vi "DAC Run.vi"(8 "error in":errorcluster, 11 "DAC HeatFlow Temp in":refnum<class "DAC HeatFlow Temp.lvclass">) -> (0 "error out":errorcluster, 3 "DAC HeatFlow Temp out":refnum<class "DAC HeatFlow Temp.lvclass">)   [LabVIEW 2019, in "DAC.lvlib" / "DAC HeatFlow Temp.lvclass"]
uses:
  DAC HeatFlow Temp.lvclass
  C:/Users/krio/Documents/LV_Projects/test-stand/App/DAC/DAC.lvclass
  DAC.lvclass/DAC.ctl
  DAC HeatFlow Temp.lvclass/DAC HeatFlow Temp.ctl
  <vilib>/DAQmx/miscellaneous.llb/DAQmx Fill In Error Info.vi
  DAC.lvclass
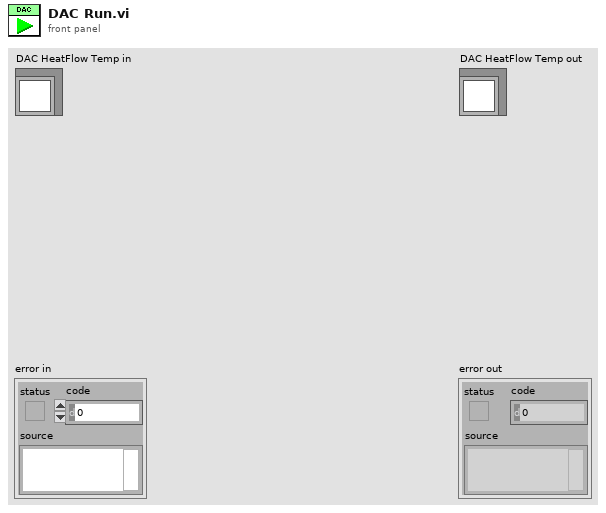
[diagram p1: front panel]
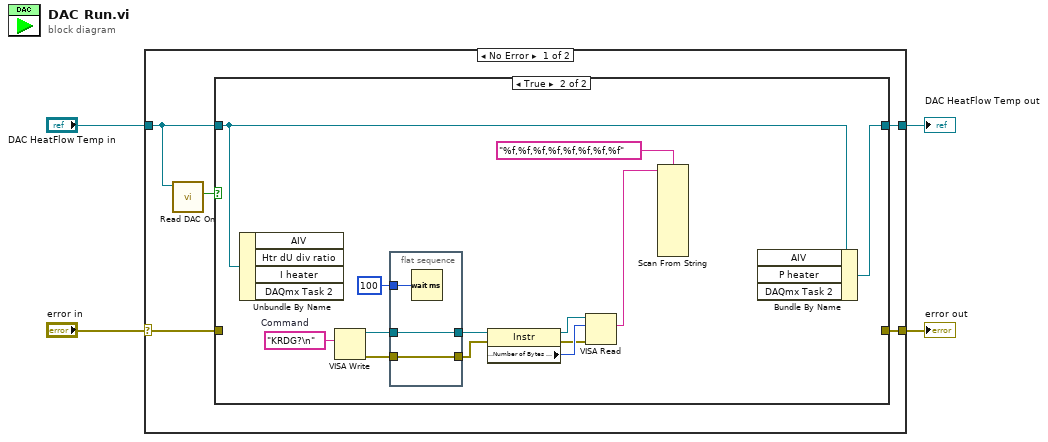
[diagram p0: block diagram]
diagram:
  n1 = case shown="No Error" "error in" {
    selector: "error in" -> [w7 w29]
    tunnel: [w6 w29] -> w2
    tunnel: [w8 w28] -> w1
    tunnel: "DAC HeatFlow Temp in" -> [w5 w28]
    frame No Error {
      n2 = call "Read DAC On.vi"("DAC in"=w5) -> ("DAC On"=w9:bool)  [unwired: 8 in, 2 out]
      n3 = case shown="True" w9 {
        tunnel: w5 -> [w11 w23]
        tunnel: [w11 w24] -> w8
        tunnel: w7 -> [w10 _]
        tunnel: [w10 _] -> w6
        frame False {
        }
        frame True {
          w22 = "KRDG?\n"  # Command
          n4 = Unbundle By Name(w23) -> ()  [unwired: 4 out]
          n5 = VISA Write(write buffer=w22) -> (VISA resource name out=w19:refnum<visa-resource-name>, error out=w20:errorcluster)  [unwired: 2 in, 1 out]
          n6 = flat-sequence {
            tunnel: u32 100 ("milliseconds to wait") -> [w27]
            tunnel: w20 -> [w26]
            tunnel: [w26] -> w17
            tunnel: w19 -> [w25]
            tunnel: [w25] -> w18
            frame #0 {
              n7 = Wait (ms)(milliseconds to wait=w27) -> ()  [unwired: 1 out]
            }
          }
          n8 = property class="Instr"(reference=w18, error in=w17) -> (reference out=w16:refnum<visa-resource-name>, error out=w14:errorcluster, "Serial Settings:Number of Bytes at Serial Port"=w15:u32)
          n9 = VISA Read(VISA resource name=w16, byte count=w15, error in (no error)=w14) -> (read buffer=w13:string)  [unwired: 3 out]
          n10 = Scan From String(format string="%f,%f,%f,%f,%f,%f,%f,%f", input string=w13) -> ()  [unwired: 18 in, 3 out]
          n11 = Bundle By Name(cluster=w23) -> (w24:refnum<class "DAC HeatFlow Temp.lvclass">)  [unwired: 3 in]
        }
      }
    }
    frame Error {
    }
  }
  "error out" <- w2
  "DAC HeatFlow Temp out" <- w1
